vi "rename.single.title.vi"(7 "index":i32, 10 "title":string, 11 "comic jsons":T1[](array[typedef])) -> (3 "comic jsons 2":T1[](array[typedef]))   [LabVIEW 2024]
uses:
  TypeDefs/comic--cluster.ctl
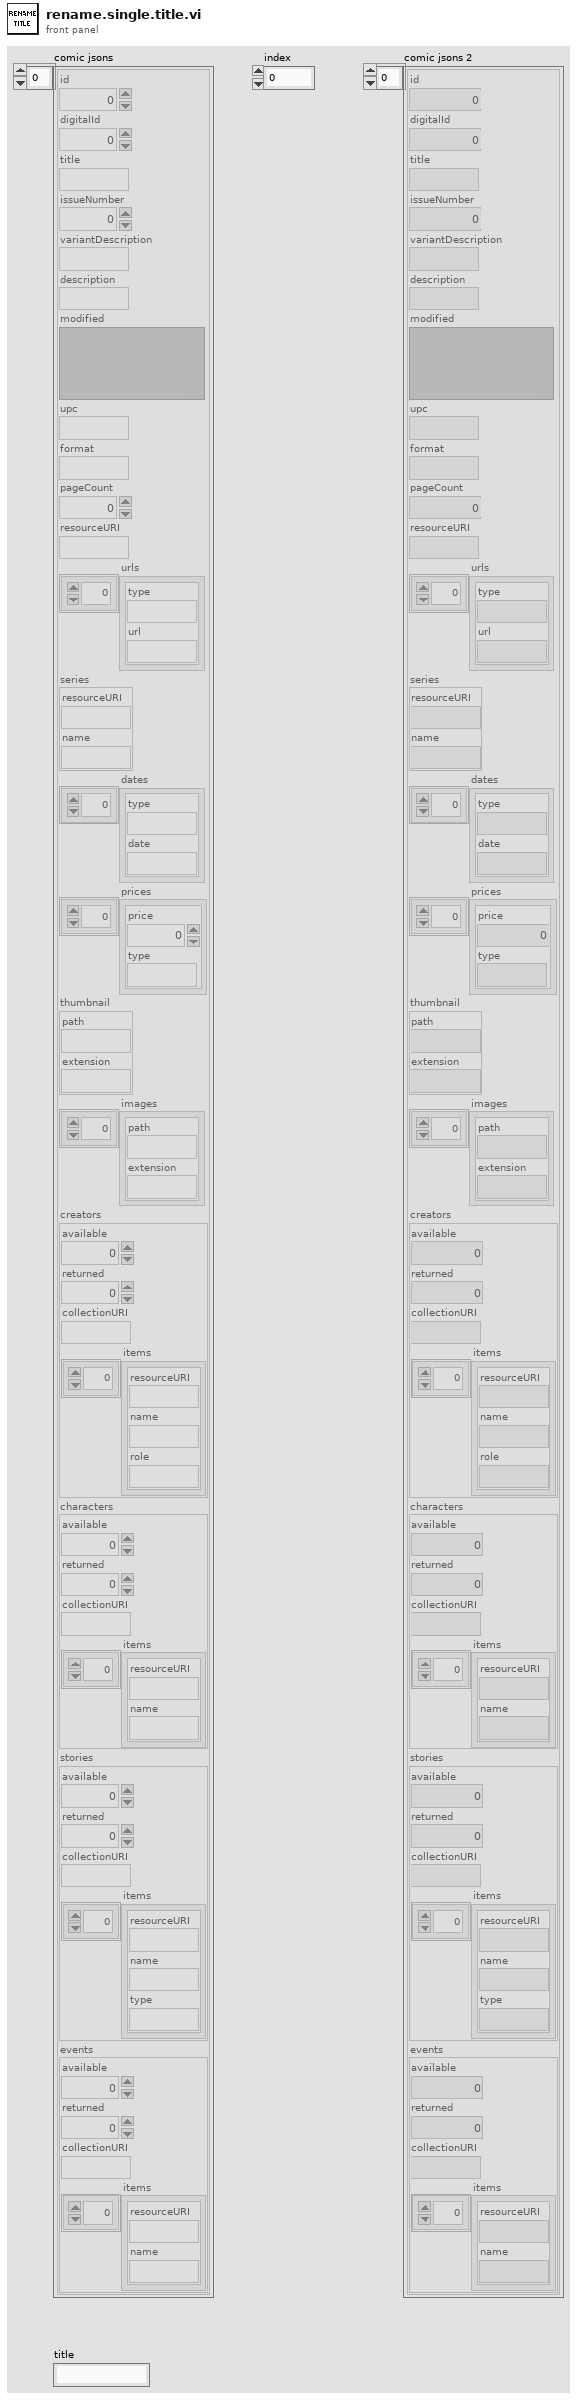
[diagram p1: front panel]
types:
  T1 = typedef "comic--cluster.ctl" = cluster{"id":i32, "digitalId":i32, "title":string, "issueNumber":i32, "variantDescription":string, "description":string, "modified":variant, "upc":string, "format":string, "pageCount":i32, "resourceURI":string, "urls":cluster{"type":string, "url":string}[], "series":cluster{"resourceURI":string, "name":string}, "dates":cluster{"type":string, "date":string}[], "prices":cluster{"price":dbl, "type":string}[], "thumbnail":cluster{"path":string, "extension":string}, "images":cluster{"path":string, "extension":string}[], "creators":cluster{"available":i32, "returned":i32, "collectionURI":string, "items":cluster{"resourceURI":string, "name":string, "role":string}[]}, "characters":cluster{"available":i32, "returned":i32, "collectionURI":string, "items":cluster{"resourceURI":string, "name":string}[]}, "stories":cluster{"available":i32, "returned":i32, "collectionURI":string, "items":cluster{"resourceURI":string, "name":string, "type":string}[]}, "events":cluster{"available":i32, "returned":i32, "collectionURI":string, "items":cluster{"resourceURI":string, "name":string}[]}}
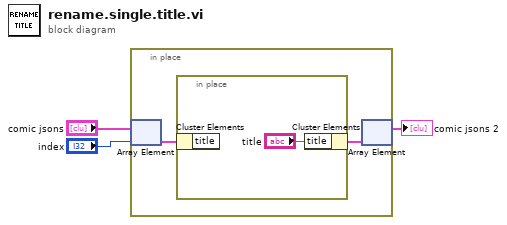
[diagram p0: block diagram]
diagram:
  n1 = in-place {
    n2 = in-place-array #1("comic jsons", "index") -> (w5:T1)
    n3 = in-place {
      n4 = in-place-cluster #2(w5) -> ()  [unwired: 1 out]
      n5 = in-place-cluster #2("title"="title") -> (w4:T1)
    }
    n6 = in-place-array #1(w4) -> (→"comic jsons 2":T1[])  [unwired: 1 out]
  }
